vi "SetParameter.vi"(8 "error in":errorcluster, 10 "value":string, 11 "Parameter":string) -> (0 "error out":errorcluster)   [LabVIEW 2013]
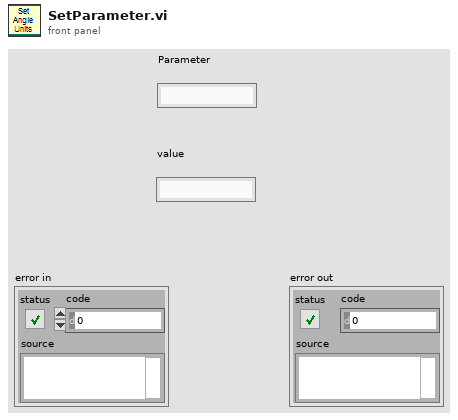
[diagram p1: front panel]
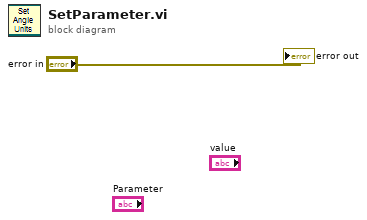
[diagram p0: block diagram]
diagram:
  "error out" <- "error in"
